vi "RTEH Display Options to Saved Options.vi"(2 "Display Error Options":T3={"Code"="", "Shared Options"={"Number of Retries"=0, "Retry"=FALSE, "Classify Output"=FALSE, "Classify Notification"=FALSE, "Convert Output to Warning"=FALSE, "Clear Output"=FALSE, "Notify"=FALSE, "Priority"=0, "Detect Warning"=FALSE, "Skip if Busy"=FALSE}, "Output Classification"="NONE", "Notification Classification"="NONE"}, 3 "Code":i32) -> (0 "Saved Error Options":T1)   [LabVIEW 2017]
uses:
  Controls/RTEH/RTEH Error Display Options.ctl
  Controls/RTEH/RTEH Shared Error Options.ctl
  Controls/RTEH/RTEH Error Options.ctl
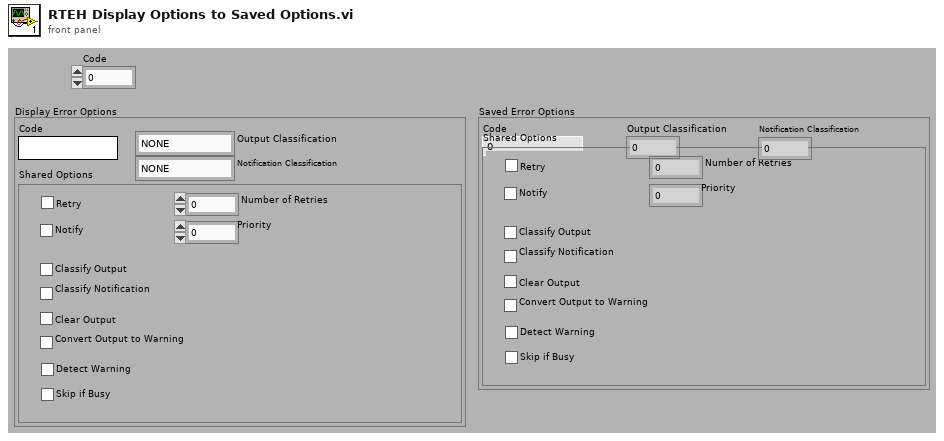
[diagram p1: front panel]
types:
  T1 = typedef "RTEH Error Options.ctl" = cluster{"Code":i32, "Shared Options":T2, "Output Classification":u32, "Notification Classification":u32}
  T2 = typedef "RTEH Shared Error Options.ctl" = cluster{"Number of Retries":i32, "Retry":bool, "Classify Output":bool, "Classify Notification":bool, "Convert Output to Warning":bool, "Clear Output":bool, "Notify":bool, "Priority":i32, "Detect Warning":bool, "Skip if Busy":bool}
  T3 = typedef "RTEH Error Display Options.ctl" = cluster{"Code":string, "Shared Options":T2, "Output Classification":string, "Notification Classification":string}
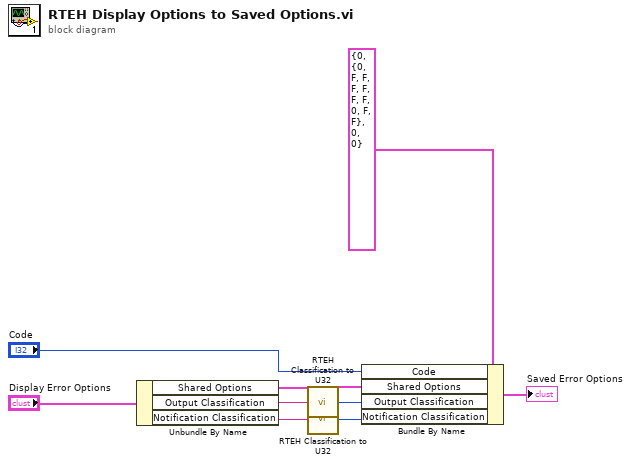
[diagram p0: block diagram]
diagram:
  n1 = Unbundle By Name("Display Error Options") -> ("Shared Options"=w6:T2, "Output Classification"=w4:string, "Notification Classification"=w2:string)
  n2 = call "RTEH Classification to U32.vi"("Classification as String"=w4) -> ("Classification as Number"=w3:u32)
  n3 = call "RTEH Classification to U32.vi"("Classification as String"=w2) -> ("Classification as Number"=w1:u32)
  n4 = Bundle By Name(cluster=T1 {"Code"=0, "Shared Options"={"Number of Retries"=0, "Retry"=FALSE, "Classify Output"=FALSE, "Classify Notification"=FALSE, "Convert Output to Warning"=FALSE, "Clear Output"=FALSE, "Notify"=FALSE, "Priority"=0, "Detect Warning"=FALSE, "Skip if Busy"=FALSE}, "Output Classification"=0, "Notification Classification"=0} ("Error Options"), "Code"="Code", "Shared Options"=w6, "Output Classification"=w3, "Notification Classification"=w1) -> (→"Saved Error Options":T1)
